vi "Start Listener.vi"(8 "error in (no error)":errorcluster, 11 "RemoteControl.STM in":refnum<class "RemoteControl.STM.lvclass">) -> (0 "error out":errorcluster, 3 "RemoteControl.STM out":refnum<class "RemoteControl.STM.lvclass">)   [LabVIEW 2019, in "RemoteControl.STM.lvclass"]
uses:
  RemoteControl.STM.lvclass
  RemoteControl.STM.lvclass/RemoteControl.STM.ctl
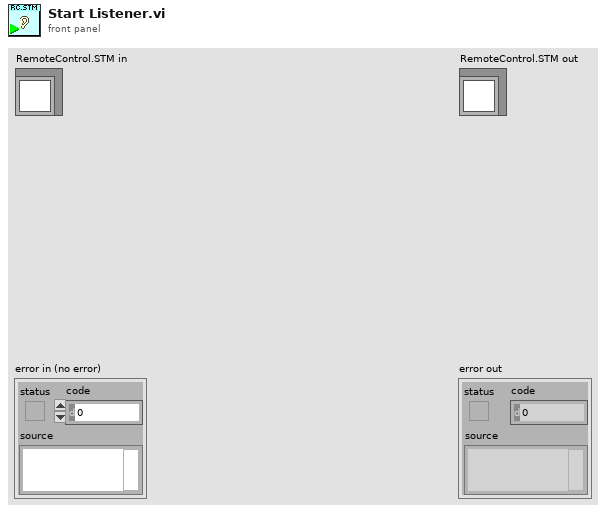
[diagram p1: front panel]
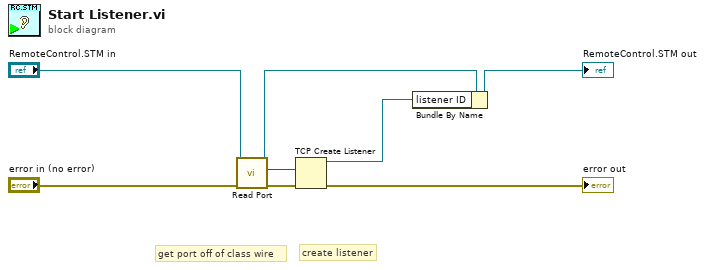
[diagram p0: block diagram]
diagram:
  # "get port off of class wire"
  # "create listener"
  n1 = call-dynamic "Read Port.vi"("error in (no error)"="error in (no error)", "RemoteControl in"="RemoteControl.STM in") -> ("error out"=w6:errorcluster, "Port"=w7:u16, "RemoteControl out"=w1:refnum<class "RemoteControl.STM.lvclass">)  [unwired: 7 in]
  n2 = TCP Create Listener(8:w6, 10:w7) -> (0:→"error out":errorcluster, 3:w8:refnum<k5>)  [unwired: 3 in, 1 out]
  n3 = Bundle By Name(cluster=w1, "listener ID"=w8) -> (→"RemoteControl.STM out":refnum<class "RemoteControl.STM.lvclass">)
